vi "CTL_SimPumpResponse.vi"(8 "Drain":bool, 9 "Fill":bool, 10 "Pump Speed":enum16{"FAST", "SLOW", "CREEP", "STOP"}(ring), 11 "PV IN":dbl) -> (3 "PV Out":dbl)   [LabVIEW 2024]
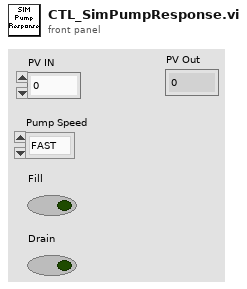
[diagram p1: front panel]
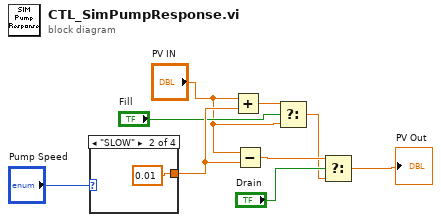
[diagram p0: block diagram]
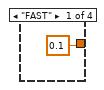
[diagram p2: hidden frame]
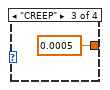
[diagram p3: hidden frame]
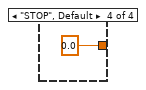
[diagram p4: hidden frame]
diagram:
  n1 = case shown="\"SLOW\"" "Pump Speed" {
    tunnel: [0.1 0.01 0.0005 0.0] -> w8
    frame "FAST" {
    }
    frame "SLOW" {
    }
    frame "CREEP" {
    }
    frame "STOP", Default {
    }
  }
  n2 = Add(x="PV IN", y=w8) -> (x+y=w7:dbl)
  n3 = Subtract(x="PV IN", y=w8) -> (x-y=w4:dbl)
  n4 = Select(t=w7, s="Fill", f="PV IN") -> (s? t:f=w2:dbl)
  n5 = Select(t=w4, s="Drain", f=w2) -> (s? t:f=→"PV Out":dbl)
